vi "dvp Vi Get Dscam Version.vi"(9 "nLength":u32, 10 "DscamVersion":string, 11 "handle":u32) -> (2 "DscamVersion out":string, 3 "function return":u32(ring))   [LabVIEW 2018, in "LabViewDVPCamera.lvlib"]
doc: "LabviewDvp2Api dvpStatus dvpViGetDscamVersion(dvpHandle handle, char *DscamVersion, dvpUint32 nLength);"
uses:
  LabViewDVPCamera.lvlib
  LabViewDVPCamera/LabViewDVPCamera.dll
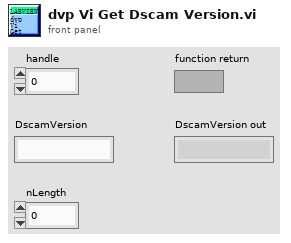
[diagram p1: front panel]
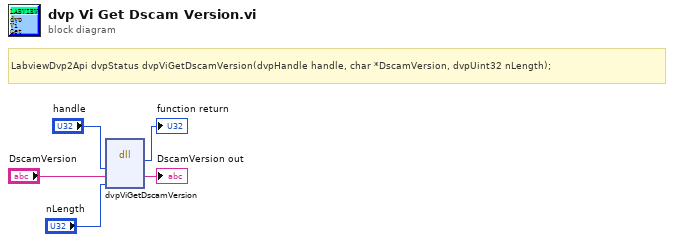
[diagram p0: block diagram]
diagram:
  # "LabviewDvp2Api dvpStatus dvpViGetDscamVersion(dvpHandle handle, char *DscamVersion, dvpUint32 nLength);"
  n1 = dll-call lib="C:/Program Files (x86)/DVP2 Labview cn 64/Sample/LabViewDVPCamera/LabViewDVPCamera.*" fn="dvpViGetDscamVersion"("handle"="handle", "DscamVersion"="DscamVersion", "nLength"="nLength") -> (→"function return":u32, "DscamVersion"=→"DscamVersion out":string)  [unwired: 5 in, 2 out]
